vi "judgeovtmsutra.vi"(0 "object in":refnum<class "interface.lvclass">, 1 "QN":string, 2 "数据输入":string, 5 "error in (no error)":errorcluster) -> (14 "object out":refnum<class "interface.lvclass">, 19 "error out":errorcluster)   [LabVIEW 2016, in "interface.lvclass"]
uses:
  interface.lvclass
  <vilib>/ptbypt/NI_PtbyPt.lvlib
  tcp_work_class/tcp_work.lvclass
panel:
  out "x+1":u32
  out "重发次数":dbl
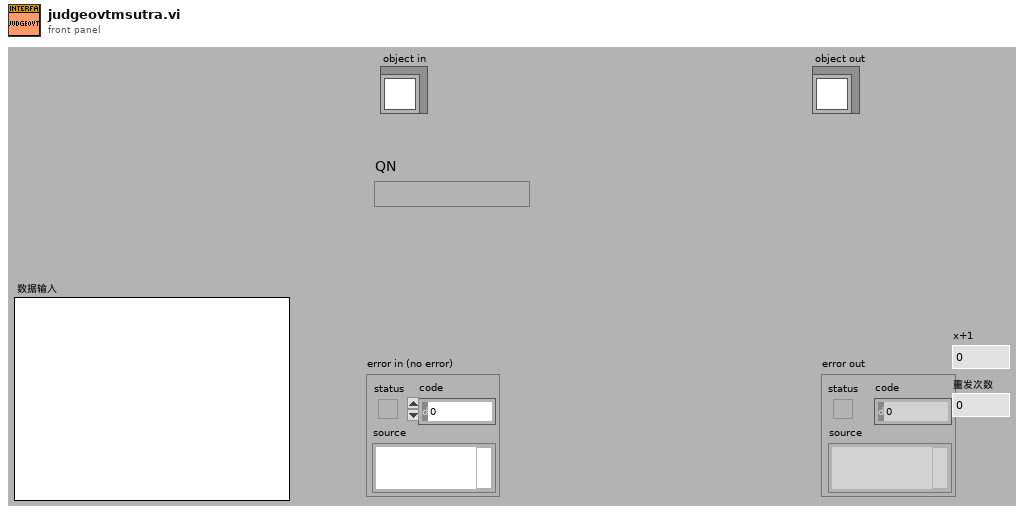
[diagram p1: front panel]
types:
  T1 = cluster{"系统状态":bool, "运行模式":bool, "测量周期":bool, "超标留样":bool, "反控数据":bool, "核查数据上传":bool, "实时小时数据上传":bool, "数据接收超时指示灯":bool, "数据发送起始时间":timestamp, "与工控软件通信":bool, "发送报文首页显示":string, "读取报文首页显示":string, "掉线指示灯":bool, "TCP掉线时间节点":string}
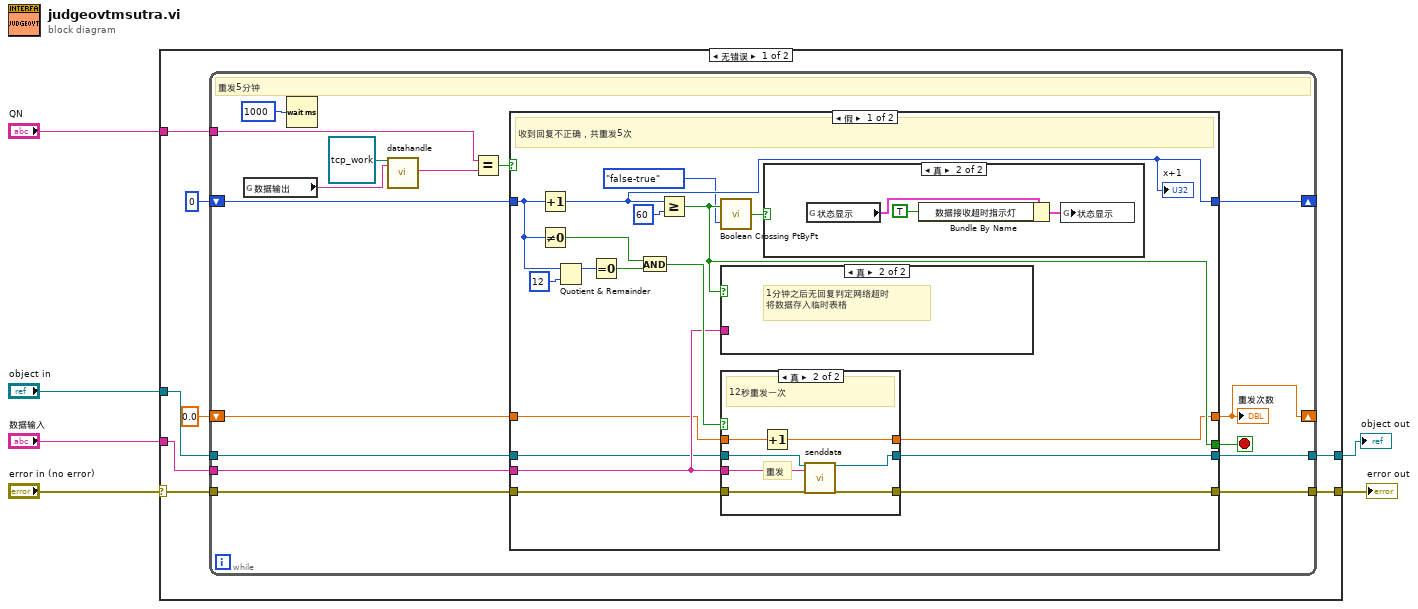
[diagram p0: block diagram]
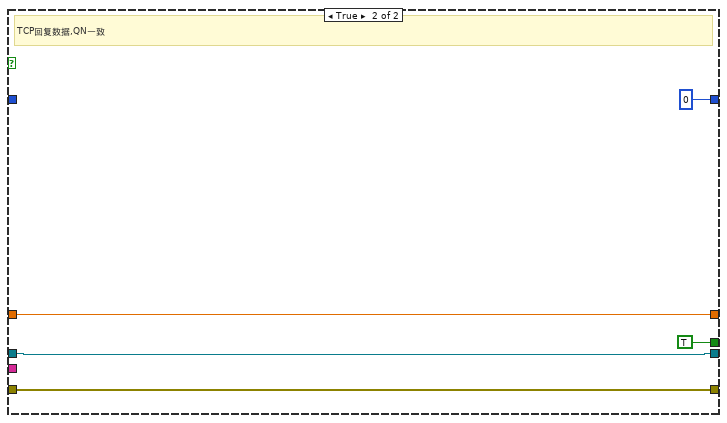
[diagram p5: hidden frame]
diagram:
  n1 = case shown="无错误" "error in (no error)" {
    selector: "error in (no error)" -> [w12 w68]
    tunnel: [w11 w68] -> w5
    tunnel: [w7 w67] -> w3
    tunnel: "object in" -> [w8 w67]
    tunnel: "数据输入" -> [w10 _]
    tunnel: "QN" -> [w9 _]
    frame No Error {
      n2 = while {
        shift-right: [w28] -> _
        shift-left: u32 0 ("等待时间（毫秒）") -> [w29]
        tunnel: [w25] -> w11
        tunnel: w10 -> [w24]
        tunnel: w12 -> [w23]
        shift-right: [w21] -> _
        shift-left: 0.0 ("重发次数") -> [w22]
        tunnel: w9 -> [w20]
        tunnel: w8 -> [w16]
        tunnel: [w15] -> w7
        stop <- w27 stop-if-true
        # "重发5分钟"
        n3 = global read "全局1.vi" "数据输出"() -> (w19:string)
        n4 = Wait (ms)(milliseconds to wait=u32 1000 ("等待时间（毫秒）")) -> ()  [unwired: 1 out]
        n5 = call-dynamic "datahandle.vi"("object in"=refnum<class "tcp_work.lvclass"> refnum ("tcp_work"), "字符串"=w19) -> ("时间QN"=w18:string)  [unwired: 12 in, 5 out]
        n6 = Equal?(x=w20, y=w18) -> (x = y?=w26:bool)
        n7 = case shown="假" w26 {
          tunnel: w29 -> [w42 _]
          tunnel: [w47 u32 0] -> w28
          tunnel: [w37 TRUE] -> w27
          tunnel: [w40 w62] -> w25
          tunnel: w24 -> [w38 _]
          tunnel: w23 -> [w39 w62]
          tunnel: w22 -> [w34 w64]
          tunnel: [w33 w64] -> w21
          tunnel: w16 -> [w32 w63]
          tunnel: [w31 w63] -> w15
          frame False {
            # "收到回复不正确，共重发5次"
            n8 = Increment(x=w42) -> (x+1=w47:u32)
            "x+1" <- w47
            n9 = Not Equal To 0?(x=w42) -> (x != 0?=w41:bool)
            n10 = Quotient & Remainder(x=w42, y=u32 12) -> (x-y*floor(x/y)=w45:u32)  [unwired: 1 out]
            n11 = Equal To 0?(x=w45) -> (x = 0?=w44:bool)
            n12 = And(x=w41, y=w44) -> (x .and. y?=w43:bool)
            n13 = Greater Or Equal?(x=w47, y=u32 60) -> (x >= y?=w37:bool)
            n14 = call <vilib>:"Boolean Crossing PtByPt.vi"("direction"=enum16{"either", "false-true", "true-false"}."false-true", "input"=w37) -> ("crossing"=w35:bool)  [unwired: 1 in]
            n15 = case shown="真" w37 {
              tunnel: w38 -> [_ _]
              frame False {
              }
              frame True {
                # "1分钟之后无回复判定网络超时\n将数据存入临时表格"
              }
            }
            n16 = case shown="真" w43 {
              tunnel: [w54 w57] -> w40
              tunnel: w38 -> [_ w59]
              tunnel: w39 -> [w54 w58]
              tunnel: w34 -> [w53 w61]
              tunnel: [w53 w60] -> w33
              tunnel: w32 -> [w52 w56]
              tunnel: [w52 w55] -> w31
              frame False {
              }
              frame True {
                # "重发"
                # "12秒重发一次"
                n17 = Increment(x=w61) -> (x+1=w60:dbl)
                n18 = call-dynamic "senddata.vi"("object in"=w56, "发送报文"=w59, "error in (no error)"=w58) -> ("object out"=w55:refnum<class "interface.lvclass">, "error out"=w57:errorcluster)  [unwired: 15 in]
              }
            }
            n19 = case shown="真" w35 {
              frame False {
              }
              frame True {
                n20 = global read "全局1.vi" "状态显示"() -> (w50:T1)
                n21 = Bundle By Name(cluster=w50, "数据接收超时指示灯"=TRUE) -> (w51:T1)
                n22 = global write "全局1.vi" "状态显示"(w51) -> ()
              }
            }
          }
          frame True {
            # "TCP回复数据,QN一致"
          }
        }
        "重发次数" <- w21
      }
    }
    frame Error {
    }
  }
  "error out" <- w5
  "object out" <- w3
